vi "20_2.vi"() -> ()   [LabVIEW 2020]
uses:
  Tile/Tile.lvclass
  Tile/Set Tile ID.vi
  Tile/Set Tile.vi
  Tile/Get Matching Sides.vi
  <userlib>/_OpenG.lib/array/array.llb/Search 1D Array (U64)__ogtk.vi
  <userlib>/_OpenG.lib/array/array.llb/Index 1D Array Elements (U64)__ogtk.vi
panel:
  out "sum 4":i16=1841
  out "Intensity Graph":i32[][](graph)
  out "Array 5":cluster{i32, i32}[](array[cluster])=[{1, 63}, {4, 22}, {8, 73}, {14, 6}, {14, 48}, {19, 33}, {25, 41}, {26, 1}, {31, 24}, {36, 64}, {40, 42}, {41, 70}, {44, 2}, {50, 22}, {51, 67}, {56, 54}, {58, 15}, {63, 28}, {67, 58}, {75, 27}, {78, 63}, {81, 20}, {86, 28}, {90, 50}]
  out "sum 3":i16=2201
  out "sum 2":i16=15
  out "Array 4":i16[](array[numeric])=[0, 0, 0, 24]
  out "sum":i16=24
  out "Array 3":bool[][](array[boolean])=[[TRUE, TRUE, TRUE, TRUE, TRUE, TRUE, TRUE, TRUE, TRUE, TRUE, TRUE, TRUE, TRUE, TRUE, TRUE, TRUE, TRUE, TRUE, FALSE, TRUE], [FALSE, TRUE, TRUE, TRUE, TRUE, FALSE, FALSE, TRUE, TRUE, TRUE, TRUE, FALSE, FALSE, TRUE, TRUE, TRUE, TRUE, FALSE, FALSE, FALSE], [TRUE, FALSE, TRUE, TRUE, FALSE, TRUE, TRUE, FALSE, TRUE, TRUE, FALSE, TRUE, TRUE, FALSE, TRUE, TRUE, FALSE, TRUE, TRUE, TRUE]]
  out "Array 2":bool[][](array[boolean])
  out "Matches 3":u64[](array[numeric])=[2789, 0, 0, 2087]
  out "Matches 2":u64[](array[numeric])=[2789, 0, 0, 2087]
  out "Array":i32[][](array[numeric])=[[1153, 1087, 2711, 2609, 1009, 2767, 1709, 1873, 2017, 2311, 2129, 1619], [2647, 3121, 1301, 1831, 3691, 1453, 3083, 1973, 2687, 1151, 3301, 1601], [3023, 3313, 1117, 2161, 1277, 3413, 1013, 2281, 2297, 1913, 1801, 3343], [2377, 3539, 1039, 1559, 2089, 1637, 1321, 1097, 3361, 1283, 2203, 2239], [3709, 3089, 3049, 2503, 2887, 1693, 1217, 3919, 2447, 3187, 1543, 3137], [2063, 1901, 2843, 3167, 3079, 2927, 2543, 3929, 3061, 2411, 1597, 2081], [1583, 2801, 2591, 1579, 2963, 1979, 3251, 3529, 1759, 2003, 1201, 1489], [3433, 3907, 3613, 3823, 3217, 3359, 2837, 2399, 1607, 1499, 2207, 1307], [1823, 3347, 2957, 3547, 2237, 3037, 2897, 2551, 2659, 3673, 1987, 3331], [3989, 3733, 1663, 1069, 3571, 1747, 2657, 3329, 1481, 1381, 2437, 1171], [3389, 3803, 3163, 2777, 1487, 3019, 3659, 3259, 3863, 2969, 3821, 2789], [3881, 2053, 3779, 2557, 2621, 1459, 2287, 1423, 1361, 2153, 2087, 1163]]
  out "Matches":u64[](array[numeric])=[1087, 2647, 0, 0]
  out "product":u64=8425574315321
  out "elements":u64[](array[numeric])=[1153, 1163, 1619, 3881]
  in  "Switch":bool
  in  "Input":string="Tile 3571:\n##..##....\n..##..#..#\n#...##....\n.....#...#\n..........\n...###....\n#......##.\n#...#...#.\n#...##...#\n#.####.##.\n\nTile 2687:\n#..##..###\n..........\n.....##..#\n.#.#..##.#\n#.#..#..##\n#.....#...\n#...#.....\n##....##..\n#...#...##\n..#.#.#.##\n\nTile 3049:\n##.#.#.###\n....##.###\n....##....\n#.........\n#.#...#..#\n#..##....#\n#.#......#\n#..#..##..\n#......###\n#.#..#...#\n\nTile 1597:\n###..##...\n##.....###\n.#..#..#.#\n#.......#.\n#.#.......\n.#..#.....\n#.....#...\n#........#\n##.#...##.\n.....#.###\n\nTile 1301:\n#.##.#.###\n#........#\n....#.....\n#.....####\n.#....#.##\n.....#....\n#..##..#.#\n.....#..##\n.#.##..#.#\n#...######\n\nTile 3259:\n..#####.#.\n.....#...#\n#...#.....\n...##...#.\n.#..#..##.\n.#.......#\n........##\n#.......#.\n.#.#...#..\n#...#.#..#\n\nTile 3989:\n#..#..####\n..........\n#........#\n.#....#...\n..........\n#.........\n.#........\n#........#\n...##.####\n.######.##\n\nTile 3803:\n#.####...#\n.###.#..#.\n....##..#.\n#........#\n..##..#...\n####.#....\n..#...#...\n#..#.....#\n..##....#.\n#....#...#\n\nTile 2897:\n.#..##.#.#\n..#.#...##\n#........#\n###.#..#.#\n...#..#.##\n...#....##\n....##...#\n.....##..#\n.#....#...\n..##....##\n\nTile 2843:\n##.###..##\n#.#.......\n#....#....\n#..##.##..\n.##..#.##.\n#....#....\n#.#...#.##\n..........\n.#...#...#\n###..#..##\n\nTile 3023:\n.#..###.#.\n.........#\n..........\n.#........\n#.#....#.#\n....#...#.\n#.......#.\n##.#.....#\n..#...#..#\n.....####.\n\nTile 2887:\n#....##...\n#...#.....\n##...##...\n#.....##.#\n.......#..\n#......#.#\n..##..#..#\n....#....#\n#.###.....\n#.####..#.\n\nTile 1013:\n#..####.#.\n#.##...#.#\n#..#..#...\n#..#..#..#\n...#......\n#.####...#\n.#..##..##\n...#.#..##\n....##..##\n#.##.#.#.#\n\nTile 3733:\n###.##.#.#\n..#....#..\n#...#.#..#\n....###..#\n.#........\n.....#....\n........##\n##........\n#........#\n#.#...#..#\n\nTile 3691:\n.##...####\n##..##....\n#.#.##..##\n#........#\n#.....##.#\n.....#....\n##.#.....#\n#..#.....#\n..#.......\n####....#.\n\nTile 3061:\n##.....#..\n.....#...#\n....##...#\n###.#.....\n#..#..###.\n#.#.###..#\n..#......#\n#..#.#...#\n..#.......\n..#.#..#..\n\nTile 1489:\n###.......\n.....##...\n..#...##..\n#.....#...\n#.#......#\n##.#..####\n...##.#...\n...#...#.#\n..........\n.##.##.#.#\n\nTile 1637:\n#########.\n.#.....#..\n#........#\n#........#\n.##.....##\n.........#\n#....#..##\n#.....####\n...###...#\n.#..##..##\n\nTile 1069:\n#.#...####\n##...#...#\n.....#...#\n.......##.\n......#..#\n#........#\n#...#.....\n......#...\n#.#..#....\n####.##.#.\n\nTile 1039:\n#..#######\n###.......\n.....#....\n#.........\n....#....#\n...####...\n.#...##...\n#.#....#.#\n........##\n#.#..#..#.\n\nTile 2767:\n.#.#..#.##\n.#..#....#\n#..#.#....\n#.#..##..#\n.####.#.##\n#....##...\n....##..##\n###.....#.\n..........\n....#.###.\n\nTile 2957:\n####.#####\n.......##.\n...#.....#\n...##..##.\n...##.##..\n#..#..#..#\n.....#....\n#..#....#.\n.##.......\n.##..#.##.\n\nTile 2789:\n.##..#.#.#\n#.#.....##\n#....#...#\n#....##...\n..#..#....\n#.........\n#.#..#..##\n#........#\n.#.......#\n#####...##\n\nTile 2837:\n.....#...#\n.....#.#.#\n#.......#.\n#...#...#.\n..#.....#.\n..#.#..#..\n##.......#\n....#....#\n#...#.....\n##.###....\n\nTile 3251:\n.######...\n...#......\n.#.#..###.\n#..#.##..#\n###.#....#\n#.#......#\n..#..###..\n##.#..#..#\n...#...###\n##.#..##..\n\nTile 3137:\n#####.#..#\n#.#..#.##.\n#.#..#....\n#.........\n.........#\n.........#\n...#......\n#...#...#.\n....#..#.#\n.#.###.#.#\n\nTile 3433:\n.##..####.\n...#......\n#..##....#\n....#....#\n#..###....\n..#......#\n.#..###...\n.##.#.....\n.........#\n.....#....\n\nTile 2551:\n#.########\n#.#.......\n##..#...##\n#.#..###.#\n#........#\n.#.#....#.\n#........#\n.##....#..\n#........#\n##..##.#..\n\nTile 2647:\n..####..##\n##....#..#\n#.........\n###.#.....\n#......#..\n....#...##\n.#..##.#.#\n.#.#..#...\n.....##.##\n.#.#...#..\n\nTile 1087:\n#..###..##\n#...#.#.#.\n.......#..\n..#.#.#..#\n#.......#.\n#....#....\n....#....#\n##...##..#\n#..#......\n.#..#.###.\n\nTile 1423:\n..#....#.#\n#........#\n.#.##.##..\n#.###.#.#.\n#.#......#\n...##...##\n#....#....\n....#....#\n.........#\n#####....#\n\nTile 1759:\n..#.#..#..\n##...#...#\n....#..#..\n#....#....\n.##..##..#\n...#.#...#\n#..#.....#\n##.......#\n......#..#\n#.##......\n\nTile 1583:\n.###.####.\n......###.\n......#..#\n.#...##...\n#...#....#\n..#.##....\n#...##..#.\n......#...\n#.....###.\n####.#....\n\nTile 1171:\n###......#\n#...##...#\n#####..##.\n#.......#.\n#.#...#..#\n#....#....\n....#....#\n##.....#.#\n#.#..#..##\n#.#.#..##.\n\nTile 2801:\n.###.####.\n......#...\n##..##.#.#\n.....#....\n#......#..\n###..##..#\n##.#..##.#\n#..#..#...\n#..#.#...#\n#..###.###\n\nTile 1559:\n.##..#...#\n#.##..#...\n...##..#..\n..#.#.....\n...#...#..\n.........#\n...#.....#\n#..##.#..#\n##..##....\n...###...#\n\nTile 2609:\n##.#..####\n..........\n#........#\n##.###...#\n#.#..#....\n..#..##..#\n#....#.#.#\n#.#.......\n#....#...#\n#.####.#.#\n\nTile 2287:\n#......#.#\n.....#.#.#\n..#..#...#\n##.#..#...\n..#..#.###\n.......###\n#......##.\n#.##.##...\n......#..#\n#####.##.#\n\nTile 3659:\n.###.#####\n#.#.......\n..........\n..#.....##\n#..#......\n#.#.#...##\n#.........\n.#...#....\n##.....#..\n#####.##.#\n\nTile 3539:\n.......#.#\n..##...#..\n.....#.#.#\n##.#......\n####......\n...#..#...\n#.......##\n#...#.....\n#..#.....#\n.##.#....#\n\nTile 3121:\n..##.#...#\n.###..#...\n##.#.#....\n#.....#..#\n#.#.......\n#.........\n....#...##\n......###.\n#........#\n#..###..##\n\nTile 2237:\n...##.....\n..........\n...#......\n#....#...#\n#.........\n.......#..\n#...###..#\n.....#...#\n.........#\n#.####.##.\n\nTile 1277:\n.###...##.\n.......###\n#.....##..\n#.##..###.\n#.#..#....\n.....#....\n#...#....#\n#.#......#\n#...###..#\n...##...##\n\nTile 2161:\n..#####..#\n#....##..#\n#.....#..#\n....#....#\n.....#.##.\n..........\n#......#.#\n#..#......\n#....#..##\n.##.....#.\n\nTile 3709:\n.#..#...##\n#..#.....#\n...#....#.\n..........\n.#...#....\n..........\n....##....\n#.........\n.........#\n..####....\n\nTile 1117:\n##.##.#..#\n.....##...\n.#.#..#.##\n.#...#..#.\n#.##.#....\n####.....#\n##..#.....\n#.........\n#...##...#\n####..#.#.\n\nTile 2081:\n##.##.###.\n#...#.....\n#.....#...\n#.#..#.#..\n#.....#..#\n...#.....#\n#....#....\n......#..#\n.#.##..#..\n###..#.#.#\n\nTile 1709:\n##...#.##.\n###..#....\n#.......#.\n#.....##..\n.........#\n#....#..##\n..#...##..\n#...#.....\n#...#.#..#\n.###.#....\n\nTile 2927:\n...###..##\n##.#......\n..........\n##........\n#....#...#\n.......##.\n#.....#..#\n##.#.#....\n#......#..\n...#.####.\n\nTile 1499:\n#....##.#.\n......#...\n#........#\n......#...\n.#.......#\n#.#...#.##\n..#....#.#\n#...#.....\n.........#\n#.....##.#\n\nTile 1453:\n#.##.####.\n..#...##..\n.........#\n.........#\n#..#..#...\n.........#\n#....#.#..\n#.....#..#\n.#........\n#....#....\n\nTile 1283:\n.#.##..###\n..#...#.#.\n...##..#..\n#.......#.\n#......#..\n#..##.....\n#.......##\n....##...#\n..#.....##\n##.#.#...#\n\nTile 2063:\n......#.##\n.........#\n....##..#.\n.#....##..\n##........\n.###.###.#\n#.#....#..\n....#...#.\n#......###\n#....####.\n\nTile 3529:\n...###.##.\n#....#...#\n...#.....#\n...#.#..#.\n.#.#.....#\n#...#.....\n##..#..#..\n#.....#..#\n.#........\n.#..#####.\n\nTile 2657:\n..#.##..#.\n##..#...##\n#.....#...\n#....##...\n.....#..##\n#.#..##.##\n#.........\n#.#...##.#\n##....#...\n##..####.#\n\nTile 2089:\n.#########\n##.#.##..#\n#........#\n#..###..##\n...#......\n##..#....#\n#...#..#..\n#..#....#.\n..#.#....#\n...###...#\n\nTile 3779:\n#.#...##.#\n.##...##..\n.....##...\n.#....##.#\n###..##..#\n#.#..#.#..\n....##...#\n##...#....\n.#...#....\n#######...\n\nTile 3217:\n...##.....\n....##....\n.....##..#\n##...#.#.#\n###.......\n...#...#..\n...#.....#\n#..#.#.###\n##.#...#.#\n.#.#..##..\n\nTile 3907:\n..#..##.##\n#.#.....##\n#.......#.\n.#...###..\n..###.####\n##.#..##..\n#.........\n##...#..#.\n#....#....\n.#.....#.#\n\nTile 3547:\n#..#.##...\n#..###...#\n##.......#\n.....#....\n#...#...#.\n#..#..#...\n........#.\n......##.#\n.......#..\n.##.#..##.\n\nTile 3187:\n##.#.##...\n#...#.##.#\n#...#.....\n#....#..##\n....#.#..#\n.....#....\n.....#..##\n....##...#\n..........\n#######.##\n\nTile 1217:\n##.#####..\n#.......#.\n...#....##\n#........#\n#.#......#\n.....#...#\n#.........\n....#...##\n#...#.....\n.#...###.#\n\nTile 3821:\n#.###.###.\n#.#......#\n#..#.#...#\n.##...#.##\n...#....##\n#...#..##.\n#......#.#\n###..#...#\n.........#\n#....##.##\n\nTile 1607:\n##..#..##.\n#.##....##\n###.##.##.\n.#....##.#\n#.#..#...#\n.....#.#..\n#.#..#..#.\n#.#..#....\n..........\n......##.#\n\nTile 1459:\n.###.##..#\n#.......#.\n##........\n..#...####\n###.......\n#....#....\n.#.....#.#\n###..#..##\n.....#....\n..#..#..##\n\nTile 2129:\n....#.#..#\n#.....##.#\n#........#\n..........\n..#......#\n#.....#..#\n.#..##...#\n#.#.#..#.#\n#.........\n#.##....##\n\nTile 1601:\n.#.#.#.#.#\n..#..##...\n#.#.#...#.\n....##....\n....##.#..\n..#.......\n#.....#..#\n#..##.#...\n.........#\n...####.#.\n\nTile 1801:\n#.#...#.#.\n..#....#..\n#..#...#..\n......#...\n.....#....\n#.#..##.##\n#.........\n...#.#...#\n.#....#..#\n#.....##..\n\nTile 2447:\n..#.....##\n.#..#...##\n.....#.#..\n.#....#..#\n#...####.#\n##.##..###\n.#.......#\n#.##.....#\n#.......##\n.###.#...#\n\nTile 2203:\n#.....##..\n#.#.......\n........##\n###...#...\n..........\n#..#.....#\n....#.##.#\n..##.....#\n.#...#...#\n#.###..#..\n\nTile 1381:\n.#...#...#\n....#.....\n##.......#\n#.....#...\n.........#\n.#.......#\n.......##.\n#.#.....##\n.#..#.##..\n##.#.##.#.\n\nTile 3163:\n#...####.#\n#......##.\n...###.#.#\n#....##...\n#......###\n.....#..##\n.#..###...\n#..##..#..\n#.....#...\n#.#####.##\n\nTile 3673:\n.#....##.#\n..#..####.\n#.....#...\n...#....#.\n#....#...#\n#....##.#.\n##...#.#..\n.#..#.#...\n#..#.....#\n####.##...\n\nTile 3919:\n....##.##.\n##..##....\n...##...##\n#...#.....\n..........\n....#..###\n.#.....#..\n....#..#.#\n.##..#....\n.#...###.#\n\nTile 2437:\n..##...#.#\n#....#...#\n#..#.....#\n..#.#...##\n.......#..\n........##\n........##\n.......#.#\n#....#.#.#\n##..#.###.\n\nTile 2969:\n##.#.##.#.\n#.##....#.\n.##......#\n#.#.#....#\n#.#.......\n.........#\n....#.#.##\n.#.......#\n...#..#.##\n##.#.##..#\n\nTile 2621:\n.##.##.#..\n.##...#...\n..........\n#.........\n#.#.#.#..#\n..#..#...#\n.......#.#\n#.#.....##\n...#..#...\n#.......##\n\nTile 3613:\n##..#....#\n#..##.....\n..#.......\n..#...#...\n...#...#..\n...#.....#\n..#.....#.\n..#.###..#\n..........\n..#.####..\n\nTile 2777:\n##.#####.#\n#.##.#...#\n..#.......\n.##...##.#\n.........#\n.#.###.##.\n#......##.\n#......##.\n#...##..##\n#..#....##\n\nTile 2711:\n#..#..##..\n..........\n#.#......#\n#.....####\n..........\n##.......#\n........#.\n#.......#.\n#.#..#...#\n#.#.####.#\n\nTile 2281:\n.#.###...#\n###....#..\n..........\n#.#..#..##\n.........#\n###..#.##.\n####..#..#\n##..#.....\n##..#..#..\n#.....#..#\n\nTile 1579:\n....#..#..\n#........#\n#...#..#..\n..##.#.#..\n.###.#...#\n....##..#.\n...##.#...\n.#.##....#\n.#.......#\n##...#...#\n\nTile 2411:\n#.#....##.\n..#...#..#\n.#..##....\n.#..##...#\n.....#.#.#\n......##..\n#.#....###\n.#.##....#\n..#..#....\n..#.###..#\n\nTile 2963:\n.......##.\n.....#....\n.........#\n#.....#..#\n.....#.#..\n.....#.##.\n.#.#...###\n#.#.......\n.#.......#\n###..#..#.\n\nTile 1693:\n#.##..##..\n..........\n.........#\n.##..#...#\n.........#\n#........#\n###......#\n..#...#...\n.#.##....#\n...#.#...#\n\nTile 2399:\n###.#.##..\n#...#.....\n...#...#.#\n###.......\n.##.##....\n##.....#.#\n####......\n##.......#\n#..#...#.#\n#...#.....\n\nTile 1913:\n##.....###\n........##\n#.....###.\n..........\n....#...#.\n#.#.....#.\n#....#...#\n..#...#...\n....#..#..\n#..####...\n\nTile 3343:\n.....#.##.\n..#...#...\n####.....#\n....#.....\n......#..#\n......#...\n#........#\n#.......#.\n..#...#.#.\n.....###.#\n\nTile 2557:\n#.......##\n....#...##\n#......#.#\n#.#.#.#.##\n#..##.....\n..###.#.#.\n#..#......\n#...#.....\n....#....#\n#.##...#.#\n\nTile 1097:\n.#.#.#..##\n..#.#.....\n##........\n.##...##..\n..#..#...#\n#........#\n........##\n#.#.#.....\n.#.#.....#\n#.##..#...\n\nTile 2591:\n##..#..###\n......#...\n...###.#..\n#.......#.\n#.#.....#.\n#.##..#...\n....##.#..\n#.#..#...#\n#.###..#.#\n##........\n\nTile 3413:\n...##...##\n..#....#..\n##.#....#.\n#..#....#.\n#........#\n#..#......\n#.....#.##\n##.....#.#\n#....#....\n####.#...#\n\nTile 2087:\n###..###.#\n##......#.\n#..#...#.#\n#.#.......\n##.#.....#\n#.#.#.....\n...#.....#\n..........\n#.........\n#.##..###.\n\nTile 3037:\n......##..\n..#..#....\n#.#.......\n#.#....#..\n.#.#.##..#\n#.....#.##\n#.....#.#.\n.#..##...#\n#....##...\n...#..###.\n\nTile 2239:\n.####..#..\n#.........\n.#.......#\n#..##.....\n##..##..##\n#.#....#..\n.........#\n#.......#.\n....#.....\n#.###..#.#\n\nTile 3313:\n##.##.#..#\n.#.#..#...\n.##...##.#\n.#.##..#..\n##........\n..........\n#..#.#....\n#.........\n..........\n.##..#..#.\n\nTile 3361:\n.###.#...#\n##..#.#..#\n...##....#\n#..##.....\n..........\n#......#.#\n.........#\n..#..##.#.\n#..#...###\n#...#.#.#.\n\nTile 3167:\n..##..####\n#.....#.#.\n.....#.#..\n...#......\n....#.#.##\n...#.#.#..\n.......#..\n##........\n#..#...#.#\n####.##..#\n\nTile 1979:\n#.#.###...\n..#.....##\n...#...##.\n#.......##\n........##\n..##..#...\n..#......#\n#.#....#.#\n#..#.....#\n.##.......\n\nTile 1831:\n##.##.##.#\n#.........\n.........#\n##.......#\n###.....##\n..##..##..\n##.....#.#\n#....#...#\n###.##..#.\n#..#####..\n\nTile 1487:\n#..#....##\n.#..#....#\n#....#....\n#.........\n#.#...#.##\n#..##...##\n...##..#..\n.#...##...\n.#........\n.#...#..#.\n\nTile 1987:\n###..#....\n##..##...#\n......#..#\n.#.#...#.#\n.....#.#..\n....#..#..\n....###..#\n#...##....\n###.....#.\n...##.####\n\nTile 3083:\n....##..#.\n##..#.###.\n#..#...##.\n#.###.....\n.........#\n....#.....\n.#........\n.#........\n#.........\n#.#.#.##.#\n\nTile 1543:\n...##..###\n.........#\n.......#.#\n#..#..#.##\n##....#.#.\n....#..#..\n#..#......\n...#...#.#\n##.##..#..\n#.###..#..\n\nTile 1151:\n#.#..#####\n#.#..#...#\n#..#......\n....#...#.\n..........\n#...#.#..#\n#..#.#...#\n##....#..#\n#.........\n##.....###\n\nTile 1009:\n##..#...##\n#....#...#\n.#...#....\n#........#\n.#..#..#..\n.###.##.#.\n#......#.#\n##.#..##..\n#....#.###\n####...##.\n\nTile 3929:\n......#.#.\n#..#.##.##\n....#.#.##\n#.##..#...\n###..#..#.\n.##..###.#\n.##......#\n....#....#\n........#.\n.#...###..\n\nTile 1321:\n#.##..#...\n.##.....##\n#.#..#....\n...#.....#\n###......#\n#.#.#.##.#\n##.......#\n##......#.\n.#...#....\n.#..##..##\n\nTile 2017:\n###.#..###\n.#..###..#\n#..#......\n.........#\n..#...##..\n....#.##.#\n...##.#..#\n....#...##\n#..#..##..\n##.#.#.#..\n\nTile 1747:\n....##.#..\n#........#\n.....#..#.\n..#####...\n######..#.\n##..#.#...\n.###..#..#\n#.....#...\n.##..#..##\n..#####...\n\nTile 3089:\n#....#.##.\n#.....#..#\n..........\n#..#.#....\n.......#..\n#.....#...\n........#.\n##..#..##.\n#.....#..#\n#.#.#....#\n\nTile 3019:\n.#..###.##\n.#...#...#\n#.#.......\n###.......\n#....#...#\n#.##...#..\n##........\n.#.......#\n.#.#......\n.#..#...#.\n\nTile 3079:\n...#.###..\n#......#..\n#.......##\n#...#..###\n#.......#.\n......#.#.\n#........#\n.#.#...###\n..#.#....#\n...#...#.#\n\nTile 1663:\n##.##..###\n#.....##.#\n......#.##\n#........#\n..#.#.....\n....#..#.#\n#.#.#..#.#\n#.......#.\n..#......#\n#.#..#....\n\nTile 1823:\n.###...###\n#.#.#..##.\n..........\n.........#\n###....#..\n..........\n##....#.##\n#.......##\n..#..#...#\n......####\n\nTile 3823:\n....#..#..\n..#.#..#.#\n###.#.##.#\n..##....#.\n#.........\n#....#...#\n#.......##\n#.#...##..\n..#....#..\n..#....##.\n\nTile 1901:\n#.#.#....#\n..#....#.#\n...#..#.#.\n.#..#..###\n....####..\n......#...\n#....#....\n..#....#..\n#......#..\n######.#..\n\nTile 3347:\n#.#.....#.\n#..#..#...\n#.#.......\n#..#.#....\n...#......\n#.........\n##.#.....#\n#........#\n#....#...#\n#.#.##.###\n\nTile 1873:\n..###.#.##\n.#.#....#.\n#........#\n..#..#...#\n##.....#..\n#........#\n#.........\n.#........\n#.#..#.#.#\n.##.#...##\n\nTile 2053:\n#.#.#.#..#\n#...###..#\n##.##.##.#\n....##.#.#\n#.###....#\n#.....#..#\n#..##.####\n....#..#..\n#.........\n#..#.#..#.\n\nTile 2659:\n.#....##.#\n#.#......#\n#..#......\n.#.###.#.#\n..........\n#........#\n.......#.#\n....#....#\n#........#\n##..##.#..\n\nTile 2503:\n.#..####.#\n#.##......\n..#....###\n..#..#.###\n...##...##\n..#.....#.\n..........\n##.#......\n#.#.......\n#...#..#.#\n\nTile 3881:\n##.###.###\n#......#..\n#...#....#\n..#.#....#\n#..#..#..#\n#..#.....#\n...#..##.#\n#.#.......\n#..##....#\n...#.##...\n\nTile 1973:\n..#.###.#.\n#.##....##\n#.......##\n##......##\n#.........\n#.#..#....\n.#....###.\n..#.#..#..\n......#..#\n#..#.....#\n\nTile 3329:\n.#.#.###.#\n..#.#.....\n.#.......#\n#..#.##.##\n#.##..####\n..#.##..##\n....#.....\n#...#.#.#.\n...#.#...#\n.#...##..#\n\nTile 3331:\n#......###\n#......#.#\n#.#.#.#..#\n........#.\n.##.####..\n#..#..#..#\n.#.......#\n......#.##\n......#.#.\n.##...#.#.\n\nTile 1307:\n##.#.#..#.\n.........#\n.#....##.#\n#.........\n#.........\n#....#.#..\n........##\n......##..\n..#.##...#\n..##...##.\n\nTile 2543:\n.#.#.##.##\n#........#\n..##......\n#.........\n##...#...#\n.###..##.#\n.##......#\n.#........\n.....#.#..\n...######.\n\nTile 2003:\n#.#..#.#.#\n.....#....\n#.#.#.....\n####.#..##\n..###....#\n....#.#...\n#.####...#\n.##...#.##\n#.#.#..#..\n...#.....#\n\nTile 3301:\n##....##.#\n.....#...#\n#........#\n..........\n###.##.#..\n.....#...#\n#.#......#\n....##...#\n#........#\n.#.#...#.#\n\nTile 2297:\n#..#.##..#\n...#.#.##.\n..###..#..\n##..#.....\n####..#..#\n..#.#..#..\n.....#...#\n#...#.....\n#.....#..#\n##....#...\n\nTile 2311:\n##.....#.#\n##........\n#........#\n#...##....\n#......#..\n.........#\n.........#\n#..#.#....\n.....#...#\n###.#..##.\n\nTile 1361:\n.#.##.#..#\n#.#..#...#\n#....###..\n..###.#...\n#..#.....#\n#..#...##.\n#.#.....#.\n.......#.#\n##.##.....\n#.###.#..#\n\nTile 1481:\n.####.#.##\n..........\n.........#\n###.#.#...\n##....##.#\n..#...#.##\n..##.#.#..\n#.#.....##\n.......#..\n....###...\n\nTile 1153:\n.##.##..##\n###......#\n#....##...\n......#.#.\n#....#....\n.....##..#\n.....#...#\n#.........\n#...#....#\n##..#.#...\n\nTile 2153:\n#.###.#..#\n..#.##....\n..##....#.\n##...#...#\n#...#.....\n........#.\n#..##...#.\n..#.......\n#...##.#..\n#.#.#.#...\n\nTile 2377:\n.##..##.#.\n...##..#.#\n#.#.#.....\n#.##......\n#.....#..#\n#...#....#\n...##....#\n...###....\n.#.##...##\n.###.##...\n\nTile 3863:\n.##.###.##\n.......#.#\n#........#\n##.#.#...#\n##...#...#\n#...##....\n#..#..#.##\n.....#####\n##.#..###.\n....###...\n\nTile 1163:\n##..######\n#........#\n.#.#...###\n..#..#...#\n##..#...##\n#.#.......\n#.#..#....\n#..#.#....\n###..#...#\n.#####.###\n\nTile 2207:\n.#..#.#.##\n##.....#.#\n#..#.....#\n#..#....##\n.........#\n...#.....#\n#...#..#..\n..#.....##\n.....#....\n#.##.....#\n\nTile 1201:\n#.##.##..#\n#.#.......\n#..#.....#\n.###...#..\n#.#......#\n........##\n.........#\n.##....#.#\n..##.#...#\n.......###\n\nTile 1619:\n#.....#.#.\n...#.##..#\n#.....#...\n#...#.....\n#..#...#.#\n#..##.#...\n.#...#.#..\n#......##.\n#.........\n#.##...###\n\nTile 3389:\n...#..##..\n#........#\n#...#.....\n#.#....#.#\n###....#.#\n#.#....###\n#..##..#.#\n.##.#.#..#\n#...###...\n#...#....#\n\nTile 3359:\n.###..##..\n#........#\n###...#.#.\n........##\n....#..#.#\n.#.#......\n#........#\n.......#.#\n.#.....#..\n##.###....\n"
  in  "Input Test":string="Tile 2311:\n..##.#..#.\n##..#.....\n#...##..#.\n####.#...#\n##.##.###.\n##...#.###\n.#.#.#..##\n..#....#..\n###...#.#.\n..###..###\n\nTile 1951:\n#.##...##.\n#.####...#\n.....#..##\n#...######\n.##.#....#\n.###.#####\n###.##.##.\n.###....#.\n..#.#..#.#\n#...##.#..\n\nTile 1171:\n####...##.\n#..##.#..#\n##.#..#.#.\n.###.####.\n..###.####\n.##....##.\n.#...####.\n#.##.####.\n####..#...\n.....##...\n\nTile 1427:\n###.##.#..\n.#..#.##..\n.#.##.#..#\n#.#.#.##.#\n....#...##\n...##..##.\n...#.#####\n.#.####.#.\n..#..###.#\n..##.#..#.\n\nTile 1489:\n##.#.#....\n..##...#..\n.##..##...\n..#...#...\n#####...#.\n#..#.#.#.#\n...#.#.#..\n##.#...##.\n..##.##.##\n###.##.#..\n\nTile 2473:\n#....####.\n#..#.##...\n#.##..#...\n######.#.#\n.#...#.#.#\n.#########\n.###.#..#.\n########.#\n##...##.#.\n..###.#.#.\n\nTile 2971:\n..#.#....#\n#...###...\n#.#.###...\n##.##..#..\n.#####..##\n.#..####.#\n#..#.#..#.\n..####.###\n..#.#.###.\n...#.#.#.#\n\nTile 2729:\n...#.#.#.#\n####.#....\n..#.#.....\n....#..#.#\n.##..##.#.\n.#.####...\n####.#.#..\n##.####...\n##..#.##..\n#.##...##.\n\nTile 3079:\n#.#.#####.\n.#..######\n..#.......\n######....\n####.#..#.\n.#...#.##.\n#.#####.##\n..#.###...\n..#.......\n..#.###..."
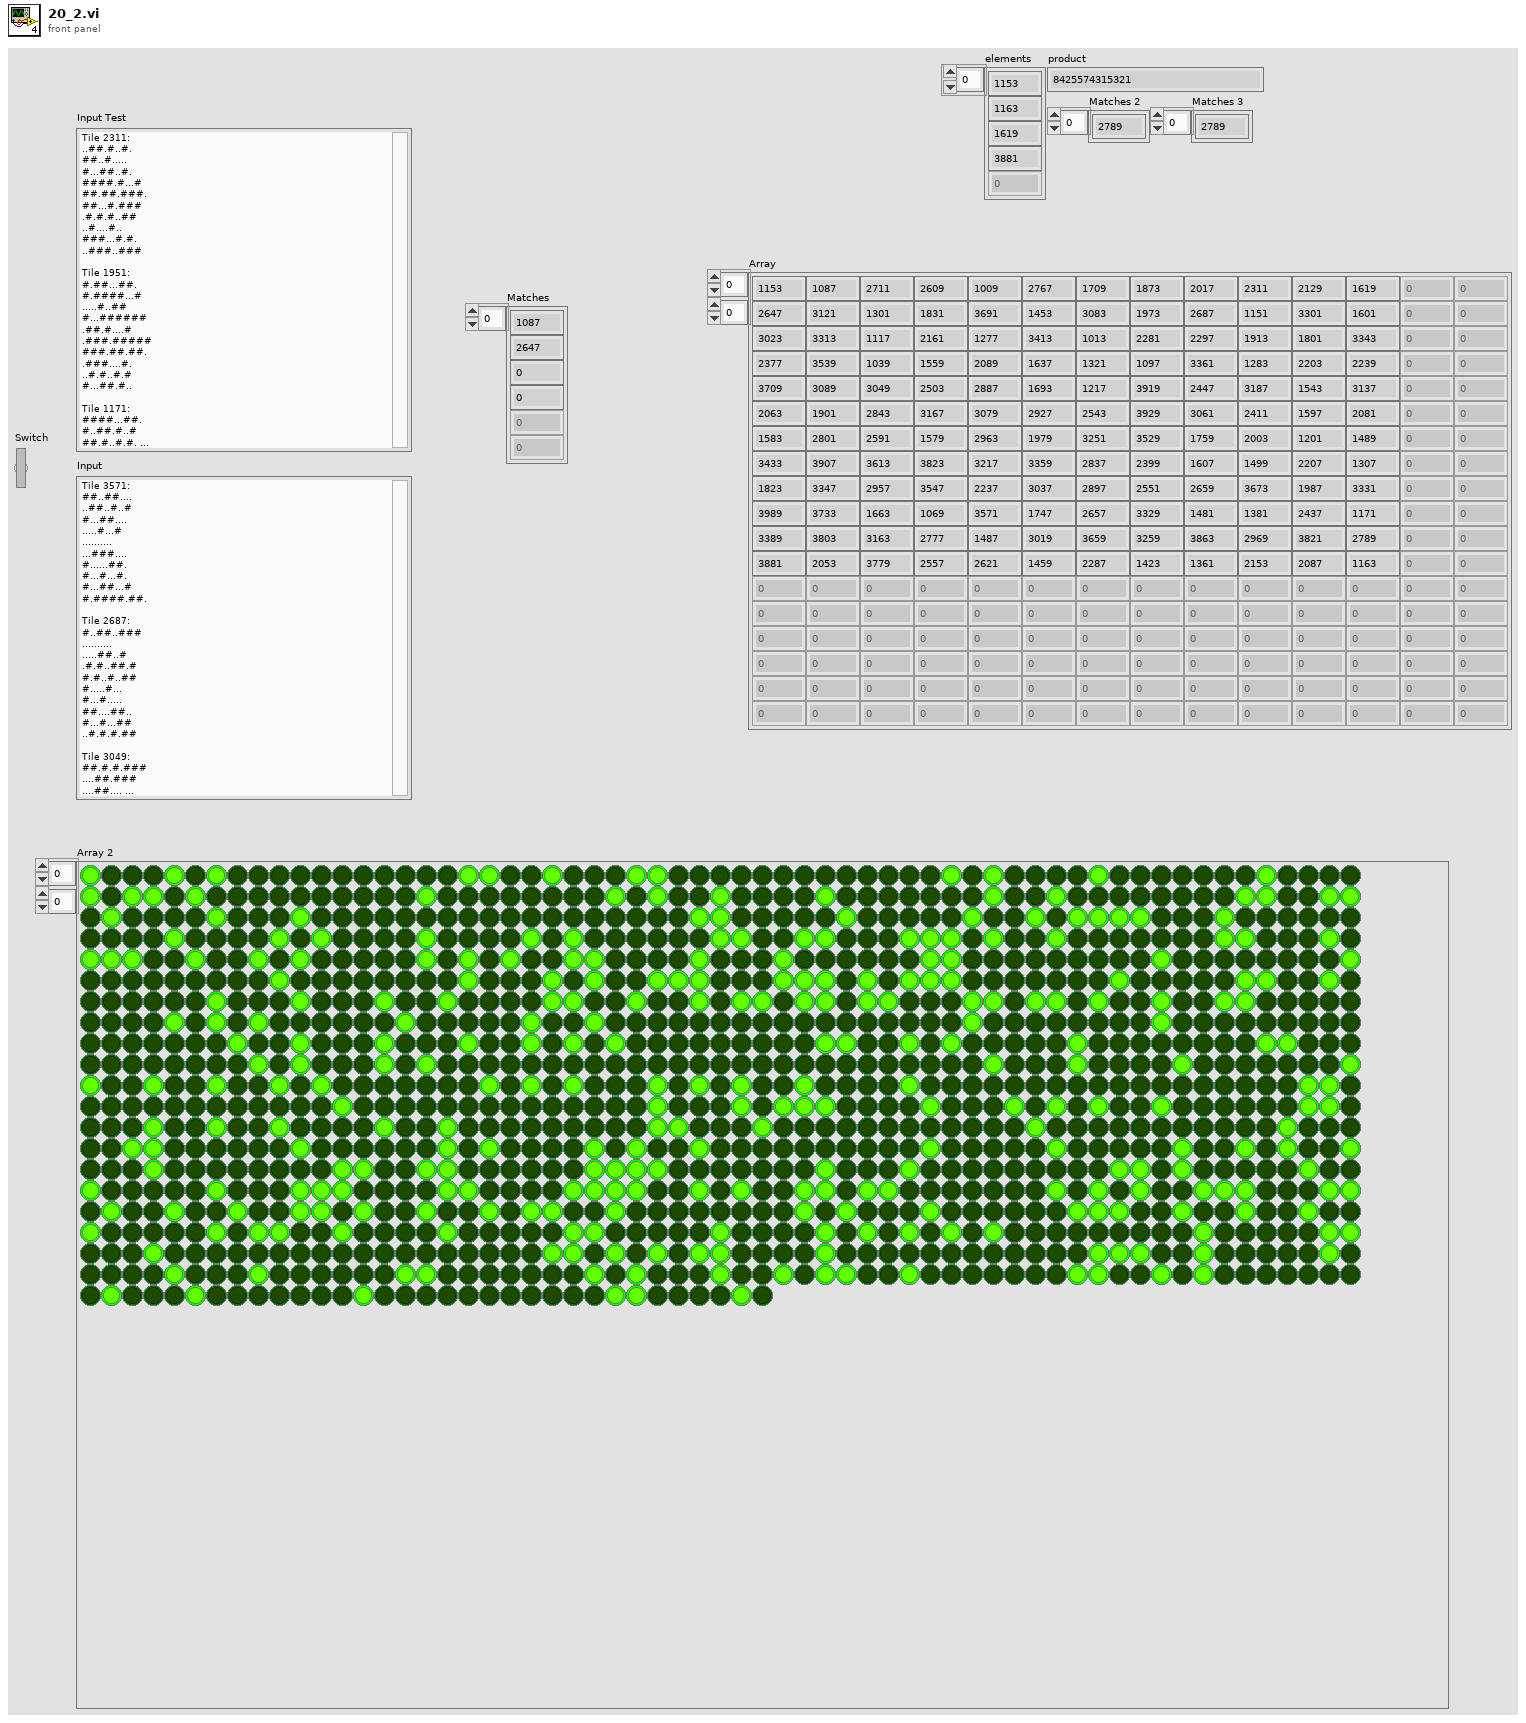
[diagram p1: front panel]
types:
  T1 = cluster{"Rotate":i32, "Flip Horizontal":bool, "Flip Vertical":bool}[]
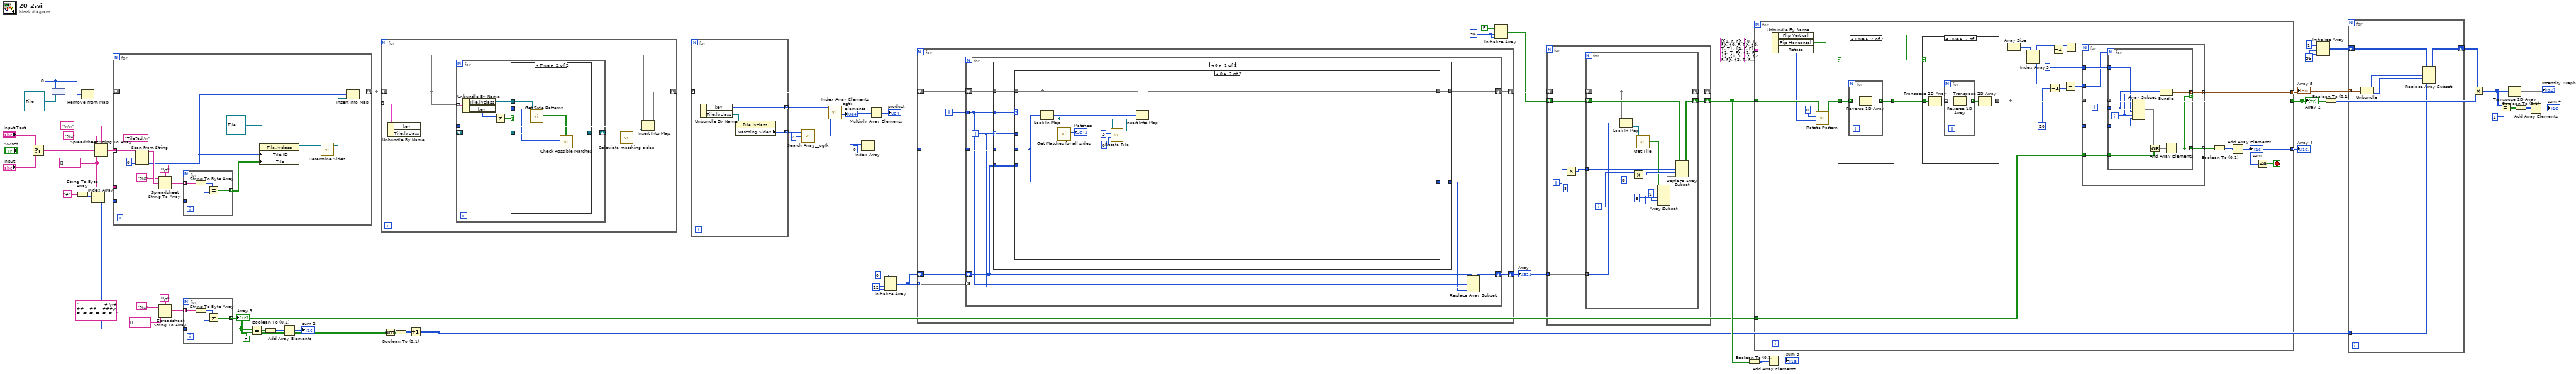
[diagram p0: block diagram]
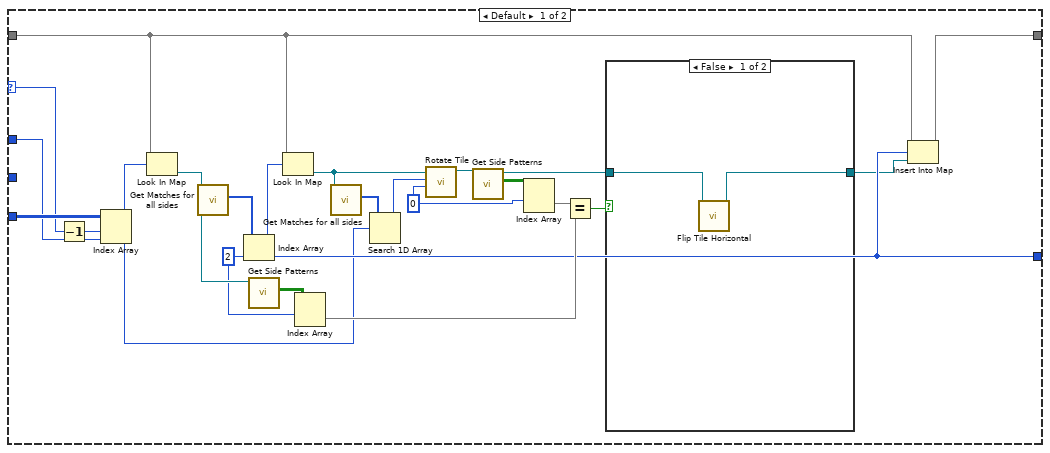
[diagram p4: hidden frame]
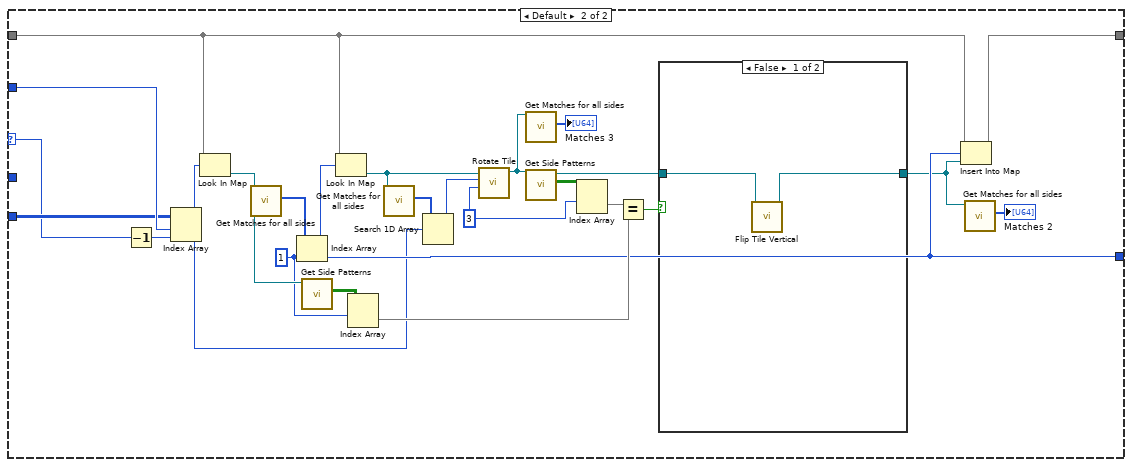
[diagram p6: hidden frame]
diagram:
  w12 = 96
  w34 = 96
  w41 = 12
  w59 = u64 0
  w55 = string[] []
  n1 = Select(t="Input Test", s="Switch", f="Input") -> (s? t:f=w51:string)
  n2 = node(w59, refnum<class "Tile.lvclass"> refnum ("Tile.lvclass")) -> (w61:map{u64, refnum<class "Tile.lvclass">})
  n3 = String To Byte Array(string="#") -> (unsigned byte array=w57:u8[])
  n4 = Remove From Map(10:w59, 11:w61) -> (3:w60:map{u64, refnum<class "Tile.lvclass">})  [unwired: 2 out]
  n5 = Index Array(array=w57) -> (element=w27:u8)  [unwired: 1 in]
  n6 = Spreadsheet String To Array(delimiter (Tab)="\n\n", format string="%s", spreadsheet string=w51, array type (2D Dbl)=w55) -> (array=w62:string[])
  n7 = for {
    tunnel: w62 -> [w78] mode=indexing
    shift-right: [w75] -> w50
    shift-left: w60 -> [w79]
    tunnel: w27 -> [w74]
    tunnel: w55 -> [w70]
    n8 = Scan From String(format string="Tile%d:\n", input string=w78, default 1=u64 0) -> (remaining string=w72:string, output 1=w65:u64)  [unwired: 2 in, 2 out]
    n9 = Spreadsheet String To Array(delimiter (Tab)="\n" ("format string"), format string="%s", spreadsheet string=w72, array type (2D Dbl)=w70) -> (array=w69:string[])
    n10 = for {
      tunnel: w74 -> [w84]
      tunnel: w69 -> [w83] mode=indexing
      tunnel: [w81] -> w68 mode=indexing
      n11 = String To Byte Array(string=w83) -> (unsigned byte array=w82:u8[])
      n12 = Equal?(x=w82, y=w84) -> (x = y?=w81:bool[])
    }
    n13 = property class="Tile.lvclass"(reference=refnum<class "Tile.lvclass"> refnum ("Tile.lvclass"), "Tile ID"=w65, "Tile"=w68) -> (reference out=w67:refnum<class "Tile.lvclass">)  [unwired: 1 in, 1 out]
    n14 = call "Determine Sides.vi"("Tile in"=w67) -> ("Tile out"=w66:refnum<class "Tile.lvclass">)  [unwired: 9 in, 1 out]
    n15 = Insert Into Map(map in=w79, key=w65, value=w66) -> (map out=w75:map{u64, refnum<class "Tile.lvclass">})  [unwired: 2 out]
  }
  n16 = Spreadsheet String To Array(delimiter (Tab)="\n" ("format string"), format string="%s", spreadsheet string="                  # \n#    ##    ##    ###\n #  #  #  #  #  #   ", array type (2D Dbl)=string[] []) -> (array=w29:string[])
  n17 = for {
    tunnel: w27 -> [w88]
    tunnel: w29 -> [w87] mode=indexing
    tunnel: [w85] -> w7 mode=indexing
    n18 = String To Byte Array(string=w87) -> (unsigned byte array=w86:u8[])
    n19 = Not Equal?(x=w86, y=w88) -> (x != y?=w85:bool[])
  }
  "Array 3" <- w7
  n20 = Equal?(x=w7, y=FALSE) -> (x = y?=w23:bool[][])
  n21 = Boolean To (0,1)(Boolean=w23) -> (0, 1=w22:i16[][])
  n22 = Add Array Elements(numeric array=w22) -> (sum=→"sum 2":i16)
  n23 = for {
    shift-right: [w94] -> w42
    shift-left: w50 -> [w92]
    tunnel: w50 -> [w95] mode=indexing
    n24 = Unbundle By Name(w95) -> ("key"=w93:u64, "Tile.lvclass"=w91:refnum<class "Tile.lvclass">)
    n25 = for {
      tunnel: w92 -> [w102] mode=indexing
      tunnel: w93 -> [w98]
      shift-right: [w96] -> w90
      shift-left: w91 -> [w97]
      n26 = Unbundle By Name(w102) -> ("Tile.lvclass"=w101:refnum<class "Tile.lvclass">, "key"=w99:u64)
      n27 = Not Equal?(x=w99, y=w98) -> (x != y?=w100:bool)
      n28 = case shown="True" w100 {
        tunnel: w101 -> [_ w108]
        tunnel: w99 -> [_ w105]
        tunnel: w97 -> [w103 w107]
        tunnel: [w103 w104] -> w96
        frame False {
        }
        frame True {
          n29 = call "Get Side Patterns.vi"("Tile in"=w108) -> ("Sides"=w106:bool[][])  [unwired: 8 in, 2 out]
          n30 = call "Check Possible Matches.vi"("Patterns In"=w106, "ID In"=w105, "Tile in"=w107) -> ("Tile out"=w104:refnum<class "Tile.lvclass">)  [unwired: 7 in, 1 out]
        }
      }
    }
    n31 = call "Calculate matching sides.vi"("Tile in"=w90) -> ("Tile out"=w89:refnum<class "Tile.lvclass">)  [unwired: 9 in, 1 out]
    n32 = Insert Into Map(map in=w92, key=w93, value=w89) -> (map out=w94:map{u64, refnum<class "Tile.lvclass">})  [unwired: 2 out]
  }
  n33 = Not(x=w7) -> (.not. x?=w17:bool[][])
  n34 = Boolean To (0,1)(Boolean=w17) -> (0, 1=w16:i16[][])
  n35 = Increment(x=w16) -> (x+1=w10:i16[][])
  n36 = for {
    tunnel: w42 -> [w112] mode=indexing
    tunnel: [w110] -> w47 mode=indexing
    tunnel: [w109] -> w49 mode=indexing
    n37 = Unbundle By Name(w112) -> ("key"=w110:u64, "Tile.lvclass"=w111:refnum<class "Tile.lvclass">)
    n38 = property class="Tile.lvclass"(reference=w111) -> ("Matching Sides"=w109:u64)  [unwired: 1 in, 2 out]
  }
  n39 = call-poly <userlib>:"Search Array__ogtk.vi"("Array"=w49, "Element Data"=u64 2 ("Matching Sides")) -> ("Indices of Elements"=w46:i32[])  [unwired: 7 in]
  n40 = call-poly <userlib>:"Index Array Elements__ogtk.vi"("indices"=w46, "array"=w47) -> ("elements"=w44:u64[])  [unwired: 9 in]
  "elements" <- w44
  n41 = Index Array(array=w44, index=0) -> (element=w39:u64)
  n42 = Multiply Array Elements(1:w44) -> (0:→"product":u64)
  n43 = Initialize Array(0, w41, w41) -> (w38:i32[][])
  n44 = for {
    tunnel: w39 -> [w113]
    shift-right: [w116] -> w37
    shift-left: w42 -> [w119]
    tunnel: w38 -> [w118] mode=indexing
    shift-right: [w114] -> w36
    shift-left: w38 -> [w115]
    i -> [w117]
    n45 = for {
      tunnel: w118 -> [_] mode=indexing
      shift-right: [w126] -> w116
      shift-left: w119 -> [w127]
      tunnel: w117 -> [w124]
      shift-right: [w122] -> w114
      shift-left: w115 -> [w120]
      tunnel: w113 -> [w125]
      i -> [w123]
      n46 = case shown="0" w123 {
        selector: w123 -> [w128 w190]
        tunnel: w127 -> [w134 w177]
        tunnel: w124 -> [w133 w192]
        tunnel: [w132 w176] -> w126
        tunnel: w125 -> [w131 _]
        tunnel: [w130 w178] -> w121
        tunnel: w120 -> [w129 w191]
        frame 0 {
          n47 = case shown="0" w133 {
            selector: w133 -> [w155 _]
            tunnel: w134 -> [w140 w161]
            tunnel: [w141 w162] -> w132
            tunnel: w131 -> [_ w163]
            tunnel: [w139 w163] -> w130
            tunnel: w129 -> [w157 _]
            tunnel: w128 -> [w156 _]
            frame Default {
              w135 = 0
              w146 = 2 ("index")
              n48 = Decrement(x=w155) -> (x-1=w154:i32)
              n49 = Index Array(array=w157, index (row)=w154, index (col)=w156) -> (element=w137:i32)
              n50 = Look In Map(map=w140, key=w137) -> (value=w148:refnum<class "Tile.lvclass">)  [unwired: 1 in, 1 out]
              n51 = call "Get Matches for all sides.vi"("Tile in"=w148) -> ("Matches"=w153:u64[])  [unwired: 8 in, 2 out]
              n52 = Index Array(array=w153, index=w146) -> (element=w139:u64)
              n53 = call "Get Side Patterns.vi"("Tile in"=w148) -> ("Sides"=w147:bool[][])  [unwired: 8 in, 2 out]
              n54 = Look In Map(map=w140, key=w139) -> (value=w151:refnum<class "Tile.lvclass">)  [unwired: 1 in, 1 out]
              n55 = Index Array(array=w147, index (row)=w146) -> (element=w144:bool[])  [unwired: 1 in]
              n56 = call "Get Matches for all sides.vi"("Tile in"=w151) -> ("Matches"=w152:u64[])  [unwired: 8 in, 2 out]
              n57 = Search 1D Array(1D array=w152, element=w137) -> (index of element=w136:i32)  [unwired: 1 in]
              n58 = call "Rotate Tile.vi"("Target"=w135, "Current"=w136, "Tile in"=w151) -> ("Tile out"=w150:refnum<class "Tile.lvclass">)  [unwired: 7 in, 1 out]
              n59 = call "Get Side Patterns.vi"("Tile in"=w150) -> ("Sides"=w149:bool[][], "Tile out"=w142:refnum<class "Tile.lvclass">)  [unwired: 8 in, 1 out]
              n60 = Index Array(array=w149, index (row)=w135) -> (element=w145:bool[])  [unwired: 1 in]
              n61 = Equal?(x=w145, y=w144) -> (x = y?=w143:bool)
              n62 = case shown="False" w143 {
                tunnel: w142 -> [w159 w160]
                tunnel: [w158 w160] -> w138
                frame False {
                  n63 = call "Flip Tile Horizontal.vi"("Tile in"=w159) -> ("Tile out"=w158:refnum<class "Tile.lvclass">)  [unwired: 9 in, 1 out]
                }
                frame True {
                }
              }
              n64 = Insert Into Map(map in=w140, key=w139, value=w138) -> (map out=w141:map{u64, refnum<class "Tile.lvclass">})  [unwired: 2 out]
            }
            frame 0 {
              n65 = Look In Map(map=w161, key=w163) -> (value=w167:refnum<class "Tile.lvclass">)  [unwired: 1 in, 1 out]
              n66 = call "Get Matches for all sides.vi"("Tile in"=w167) -> ("Matches"=→"Matches":u64[])  [unwired: 8 in, 2 out]
              n67 = call "Rotate Tile.vi"("Target"=0 ("Current"), "Current"=3, "Tile in"=w167) -> ("Tile out"=w164:refnum<class "Tile.lvclass">)  [unwired: 7 in, 1 out]
              n68 = Insert Into Map(map in=w161, key=w163, value=w164) -> (map out=w162:map{u64, refnum<class "Tile.lvclass">})  [unwired: 2 out]
            }
          }
        }
        frame Default {
          w169 = 3
          w179 = 1 ("index")
          n69 = Decrement(x=w190) -> (x-1=w193:i32)
          n70 = Index Array(array=w191, index (row)=w192, index (col)=w193) -> (element=w175:i32)
          n71 = Look In Map(map=w177, key=w175) -> (value=w185:refnum<class "Tile.lvclass">)  [unwired: 1 in, 1 out]
          n72 = call "Get Matches for all sides.vi"("Tile in"=w185) -> ("Matches"=w189:u64[])  [unwired: 8 in, 2 out]
          n73 = Index Array(array=w189, index=w179) -> (element=w178:u64)
          n74 = call "Get Side Patterns.vi"("Tile in"=w185) -> ("Sides"=w184:bool[][])  [unwired: 8 in, 2 out]
          n75 = Look In Map(map=w177, key=w178) -> (value=w187:refnum<class "Tile.lvclass">)  [unwired: 1 in, 1 out]
          n76 = Index Array(array=w184, index (row)=w179) -> (element=w182:bool[])  [unwired: 1 in]
          n77 = call "Get Matches for all sides.vi"("Tile in"=w187) -> ("Matches"=w188:u64[])  [unwired: 8 in, 2 out]
          n78 = Search 1D Array(1D array=w188, element=w175) -> (index of element=w170:i32)  [unwired: 1 in]
          n79 = call "Rotate Tile.vi"("Target"=w169, "Current"=w170, "Tile in"=w187) -> ("Tile out"=w172:refnum<class "Tile.lvclass">)  [unwired: 7 in, 1 out]
          n80 = call "Get Matches for all sides.vi"("Tile in"=w172) -> ("Matches"=→"Matches 3":u64[])  [unwired: 8 in, 2 out]
          n81 = call "Get Side Patterns.vi"("Tile in"=w172) -> ("Sides"=w186:bool[][], "Tile out"=w180:refnum<class "Tile.lvclass">)  [unwired: 8 in, 1 out]
          n82 = Index Array(array=w186, index (row)=w169) -> (element=w183:bool[])  [unwired: 1 in]
          n83 = Equal?(x=w183, y=w182) -> (x = y?=w181:bool)
          n84 = case shown="False" w181 {
            tunnel: w180 -> [w195 w196]
            tunnel: [w194 w196] -> w174
            frame False {
              n85 = call "Flip Tile Vertical.vi"("Tile in"=w195) -> ("Tile out"=w194:refnum<class "Tile.lvclass">)  [unwired: 9 in, 1 out]
            }
            frame True {
            }
          }
          n86 = Insert Into Map(map in=w177, key=w178, value=w174) -> (map out=w176:map{u64, refnum<class "Tile.lvclass">})  [unwired: 2 out]
          n87 = call "Get Matches for all sides.vi"("Tile in"=w174) -> ("Matches"=→"Matches 2":u64[])  [unwired: 8 in, 2 out]
        }
      }
      n88 = Replace Array Subset(array=w120, new element=w121, index (row)=w124, index (col)=w123) -> (w122:i32[][])
    }
  }
  "Array" <- w36
  n89 = Initialize Array(FALSE, w34, w34) -> (w33:bool[][])
  n90 = for {
    shift-right: [w201] -> _
    shift-left: w37 -> [w202]
    tunnel: w36 -> [w204] mode=indexing
    shift-right: [w197] -> w20
    shift-left: w33 -> [w203]
    i -> [w200]
    n91 = Multiply(x=w200, y=8) -> (x*y=w199:i32)
    n92 = for {
      tunnel: w204 -> [w217] mode=indexing
      shift-right: [w211] -> w197
      shift-left: w203 -> [w215]
      shift-right: [w210] -> w201
      shift-left: w202 -> [w210]
      tunnel: w199 -> [w214]
      i -> [w213]
      w206 = 8 ("index")
      w207 = 1 ("index")
      n93 = Look In Map(map=w210, key=w217) -> (value=w216:refnum<class "Tile.lvclass">)  [unwired: 1 in, 1 out]
      n94 = Multiply(x=w213, y=8) -> (x*y=w212:i32)
      n95 = call "Get Tile.vi"("Tile in"=w216) -> ("Tile"=w208:bool[][])  [unwired: 8 in, 2 out]
      n96 = Array Subset(array=w208, index (row)=w207, length (row)=w206, index (col)=w207, length (col)=w206) -> (w205:bool[][])
      n97 = Replace Array Subset(array=w215, new element=w205, index (row)=w214, index (col)=w212) -> (w211:bool[][])
    }
  }
  n98 = Boolean To (0,1)(Boolean=w20) -> (0, 1=w19:i16[][])
  n99 = for {
    tunnel: w7 -> [w241]
    tunnel: w20 -> [w238]
    tunnel: [w230] -> w25 mode=indexing
    tunnel: T1 [{"Rotate"=0, "Flip Horizontal"=FALSE, "Flip Vertical"=FALSE}, {"Rotate"=0, "Flip Horizontal"=TRUE, "Flip Vertical"=FALSE}, {"Rotate"=0, "Flip Horizontal"=FALSE, "Flip Vertical"=TRUE}, {"Rotate"=0, "Flip Horizontal"=TRUE, "Flip Vertical"=TRUE}, {"Rotate"=1, "Flip Horizontal"=FALSE, "Flip Vertical"=FALSE}, {"Rotate"=1, "Flip Horizontal"=TRUE, "Flip Vertical"=FALSE}, {"Rotate"=1, "Flip Horizontal"=FALSE, "Flip Vertical"=TRUE}, {"Rotate"=1, "Flip Horizontal"=TRUE, "Flip Vertical"=TRUE}, {"Rotate"=2, "Flip Horizontal"=FALSE, "Flip Vertical"=FALSE}, {"Rotate"=2, "Flip Horizontal"=TRUE, "Flip Vertical"=FALSE}, {"Rotate"=2, "Flip Horizontal"=FALSE, "Flip Vertical"=TRUE}, {"Rotate"=2, "Flip Horizontal"=TRUE, "Flip Vertical"=TRUE}, {"Rotate"=3, "Flip Horizontal"=FALSE, "Flip Vertical"=FALSE}, {"Rotate"=3, "Flip Horizontal"=TRUE, "Flip Vertical"=FALSE}, {"Rotate"=3, "Flip Horizontal"=FALSE, "Flip Vertical"=TRUE}, {"Rotate"=3, "Flip Horizontal"=TRUE, "Flip Vertical"=TRUE}] ("Array") -> [w234] mode=indexing
    tunnel: [w227] -> w15
    tunnel: [w229] -> w14 mode=concatenating
    stop <- w228 stop-if-true
    w219 = 20
    w225 = 3
    n100 = Unbundle By Name(w234) -> ("Flip Vertical"=w232:bool, "Flip Horizontal"=w231:bool, "Rotate"=w233:i32)
    n101 = call "Rotate Pattern.vi"("Target"=w233, "Current"=0, "Pattern In"=w238) -> ("Pattern Out"=w237:bool[][])  [unwired: 7 in, 1 out]
    n102 = case shown="True" w231 {
      tunnel: w237 -> [w242 w244]
      tunnel: [w242 w243] -> w236
      frame False {
      }
      frame True {
        n103 = for {
          tunnel: w244 -> [w246] mode=indexing
          tunnel: [w245] -> w243 mode=indexing
          n104 = Reverse 1D Array(array=w246) -> (reversed array=w245:bool[])
        }
      }
    }
    n105 = case shown="True" w232 {
      tunnel: w236 -> [w247 w251]
      tunnel: [w247 w248] -> w227
      frame False {
      }
      frame True {
        n106 = Transpose 2D Array(2D array=w251) -> (transposed array=w249:bool[][])
        n107 = for {
          tunnel: w249 -> [w253] mode=indexing
          tunnel: [w252] -> w250 mode=indexing
          n108 = Reverse 1D Array(array=w253) -> (reversed array=w252:bool[])
        }
        n109 = Transpose 2D Array(2D array=w250) -> (transposed array=w248:bool[][])
      }
    }
    n110 = Array Size(array=w227) -> (size(s)=w224:i32[])
    n111 = Index Array(array=w224) -> (element #1=w223:i32, element #2=w222:i32)  [unwired: 2 in]
    n112 = Decrement(x=w219) -> (x-1=w218:i32)
    n113 = Decrement(x=w225) -> (x-1=w220:i32)
    n114 = Subtract(x=w222, y=w218) -> (x-y=w221:i32)
    n115 = Subtract(x=w223, y=w220) -> (x-y=w226:i32)
    n116 = for {
      N: w226 -> [_]
      tunnel: w227 -> [w261]
      tunnel: w241 -> [w259]
      tunnel: [w258] -> w240 mode=concatenating
      tunnel: [w257] -> w229 mode=concatenating
      tunnel: w225 -> [w256]
      tunnel: w219 -> [w255]
      tunnel: w221 -> [w254]
      i -> [w260]
      n117 = for {
        N: w254 -> [_]
        tunnel: w261 -> [w271]
        tunnel: w260 -> [w267]
        tunnel: w259 -> [w270]
        tunnel: [w264] -> w258 mode=indexing
        tunnel: [w265] -> w257 mode=indexing if=w264
        tunnel: w256 -> [w263]
        tunnel: w255 -> [w262]
        i -> [w266]
        n118 = Array Subset(array=w271, index (row)=w267, length (row)=w263, index (col)=w266, length (col)=w262) -> (w269:bool[][])
        n119 = Or(x=w269, y=w270) -> (x .or. y?=w268:bool[][])
        n120 = Bundle(w267, w266) -> (w265:cluster{i32, i32})  [unwired: 1 in]
        n121 = And Array Elements(Boolean array=w268) -> (logical AND=w264:bool)
      }
    }
    n122 = Boolean To (0,1)(Boolean=w240) -> (0, 1=w239:i16[])
    n123 = Add Array Elements(numeric array=w239) -> (sum=w230:i16)
    "sum" <- w230
    n124 = Not Equal To 0?(x=w230) -> (x != 0?=w228:bool)
  }
  "Array 4" <- w25
  "Array 2" <- w15
  "Array 5" <- w14
  n125 = Add Array Elements(numeric array=w19) -> (sum=→"sum 3":i16)
  n126 = Initialize Array(1, w12, w12) -> (w11:i32[][])
  n127 = Boolean To (0,1)(Boolean=w15) -> (0, 1=w9:i16[][])
  n128 = for {
    tunnel: w14 -> [w277] mode=indexing
    shift-right: [w272] -> w8
    shift-left: w11 -> [w276]
    tunnel: w10 -> [w273]
    n129 = Unbundle(w277) -> (w275:i32, w274:i32)
    n130 = Replace Array Subset(array=w276, new element=w273, index (row)=w275, index (col)=w274) -> (w272:i32[][])
  }
  n131 = Multiply(x=w8, y=w9) -> (x*y=w5:i32[][])
  n132 = Equal?(x=w5, y=1) -> (x = y?=w3:bool[][])
  n133 = Transpose 2D Array(2D array=w5) -> (transposed array=→"Intensity Graph":i32[][])
  n134 = Boolean To (0,1)(Boolean=w3) -> (0, 1=w2:i16[][])
  n135 = Add Array Elements(numeric array=w2) -> (sum=→"sum 4":i16)
